vi "Write configuration.vi"(8 "error in":errorcluster, 10 "CEF Configuration":refnum<class "CEF_serializable configuration.lvclass">, 11 "HW Engine in":refnum<class "HW Engine.lvclass">) -> (0 "error out":errorcluster, 3 "HW Engine out":refnum<class "HW Engine.lvclass">)   [LabVIEW 2025, in "HW Engine.lvlib" / "HW Engine.lvclass"]
doc: "Copyright 2017 National Instruments Corporation\n\nLicensed under the Apache License, Version 2.0 (the \"License\"); you may not use this file except in compliance with the License. You may obtain a copy of the License at http://www.apache.org/licenses/LICENSE-2.0\nUnless required by applicable law or agreed to in writing, software distributed under the License is distributed on an \"AS IS\" BASIS, WITHOUT WARRANTIES OR CONDITIONS OF ANY KIND, either express or implied. See the License for the specific language governing permissions and limitations under the License."
uses:
  HW Engine.lvclass
  Users/Public/Documents/Sandia National Labs/TSS Plugin/CEF.lvlibp/serializable configuration/CEF_serializable configuration.lvclass
  HW Engine.lvclass/HW Engine.ctl
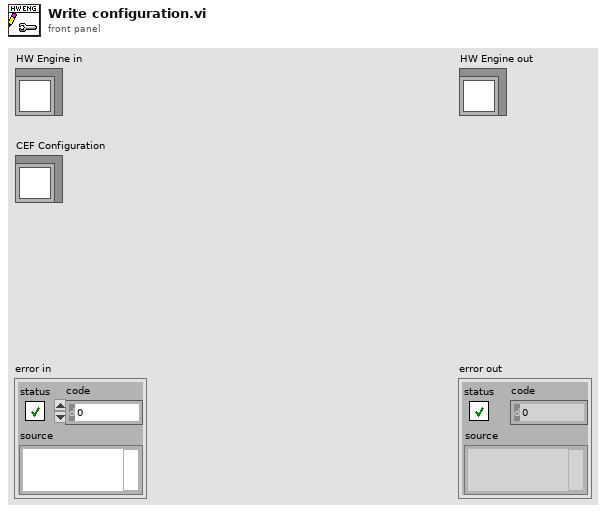
[diagram p1: front panel]
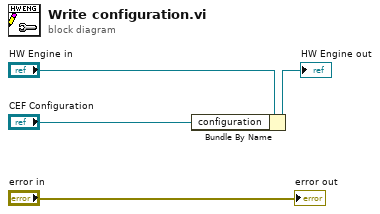
[diagram p0: block diagram]
diagram:
  n1 = Bundle By Name(cluster="HW Engine in", "configuration"="CEF Configuration") -> (→"HW Engine out":refnum<class "HW Engine.lvclass">)
  "error out" <- "error in"
